vi "myRIO_BRig_RT_dataExp_Tcycle_Reward_min_R.vi"() -> (2 "output_Tcycle_Reward_min_R":i32)   [LabVIEW 2014]
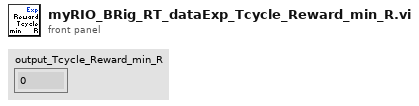
[diagram p1: front panel]
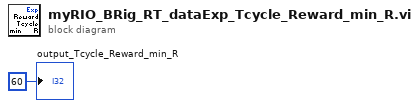
[diagram p0: block diagram]
diagram:
  "output_Tcycle_Reward_min_R" <- 60 ("output_iBlock")
